vi "initialise.vi"(8 "error in (no error)":errorcluster, 11 "DL090215DataCollection in":refnum<class "DataCollectionDL110128Streaming.lvclass">) -> (0 "error out":errorcluster, 3 "DL090215DataCollection out":refnum<class "DataCollectionDL110128Streaming.lvclass">)   [LabVIEW 2010, in "DataCollectionDL110128Streaming.lvclass"]
uses:
  DataCollectionDL110128Streaming.lvclass
  common/enumerations/top-level_component_type_enum.ctl
  DataCollectionDL091104Scaffold/DataCollectionDL091104Scaffold/DataCollectionDL091104Scaffold.lvclass
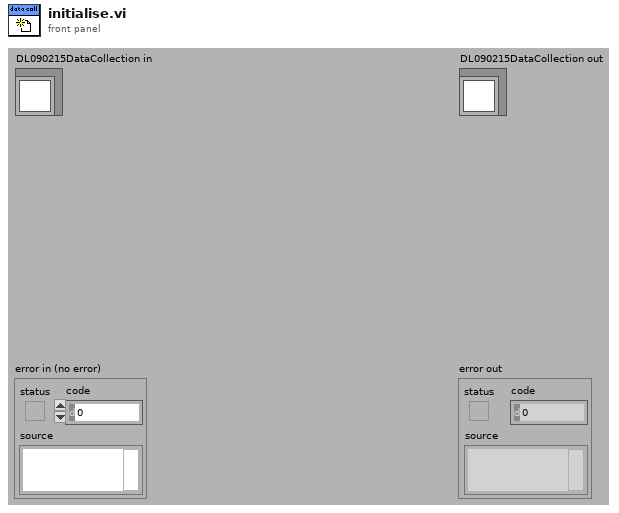
[diagram p1: front panel]
types:
  T1 = typedef "top-level_component_type_enum.ctl" = enum16{"undefined", "ImagingMode", "ScanHead", "DAQ", "ImageAssembler", "Display", "DataCollection", "Analyser", "Stimulator", "ExperimentController", "Instrument", "Stage"}
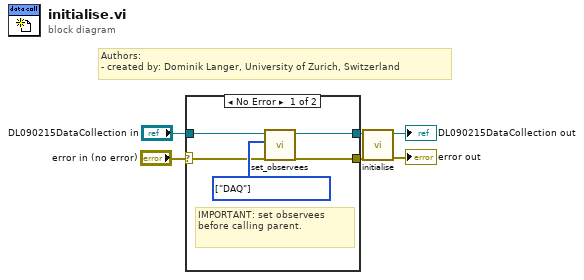
[diagram p0: block diagram]
diagram:
  # "Authors: \n- created by: Dominik Langer, University of Zurich, Switzerland"
  n1 = case shown="No Error" "error in (no error)" {
    selector: "error in (no error)" -> [w7 w12]
    tunnel: [w11 w12] -> w4
    tunnel: "DL090215DataCollection in" -> [w9 w13]
    tunnel: [w8 w13] -> w2
    frame No Error {
      w10 = T1[] [enum."DAQ"] items=["undefined", "ImagingMode", "ScanHead", "DAQ", "ImageAssembler", "Display", "DataCollection", "Analyser", "Stimulator", "ExperimentController", "Instrument", "Stage"] ("observees")
      # "IMPORTANT: set observees before calling parent."
      n2 = call-dynamic "set_observees.vi"("error in (no error)"=w7, "observees"=w10, "GenericToplevelComponent in"=w9) -> ("error out"=w11:errorcluster, "GenericToplevelComponent out"=w8:refnum<class "DataCollectionDL110128Streaming.lvclass">)  [unwired: 7 in]
    }
    frame Error {
    }
  }
  n3 = call-parent "initialise.vi"("error in (no error)"=w4, "DL090215DataCollection in"=w2) -> ("error out"=→"error out":errorcluster, "DL090215DataCollection out"=→"DL090215DataCollection out":refnum<class "DataCollectionDL110128Streaming.lvclass">)  [unwired: 8 in]
